vi "Test Read Strings.vi"(11 "TwinCAT ADS in":refnum<class "TwinCAT ADS.lvclass">) -> (3 "TwinCAT ADS out":refnum<class "TwinCAT ADS.lvclass">)   [LabVIEW 2018]
uses:
  TwinCAT ADS Class/TwinCAT ADS.lvclass
  da5912db-239c-466c-8894-2e4d3d3515d5.vi
  0b8e16e0-dc07-46b7-b0c9-e61de058ac04.vi
  9020aa95-6034-4dbf-83dd-b9edd1e76234.vi
  e5c40106-6d15-478c-83d1-da726149c43f.vi
  d432d6b6-cb13-4d15-9f79-374da6932203.vi
  66708433-c380-4caa-81db-290be98b0d9d.vi
  0e82c4fa-873b-4361-ac99-2e6e4b7cd392.vi
  da0f88be-82f8-4e5b-86e7-5baa69d9b51e.vi
  4782b519-43e7-4b8e-bd72-e209be860882.vi
  e7a7b24b-aede-49d7-b369-bb451e1de87e.vi
  TwinCAT ADS Class/VIs/Data/Read.vi
  <vilib>/addons/_JKI Toolkits/Caraya/classes/Assert/Assert Equal Value and Type_Variant.vi
  <vilib>/addons/_JKI Toolkits/Caraya/classes/Assert/Assert.lvclass
  <vilib>/addons/_JKI Toolkits/Caraya/classes/Test/Test.lvclass
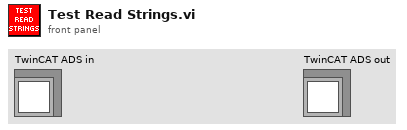
[diagram p1: front panel]
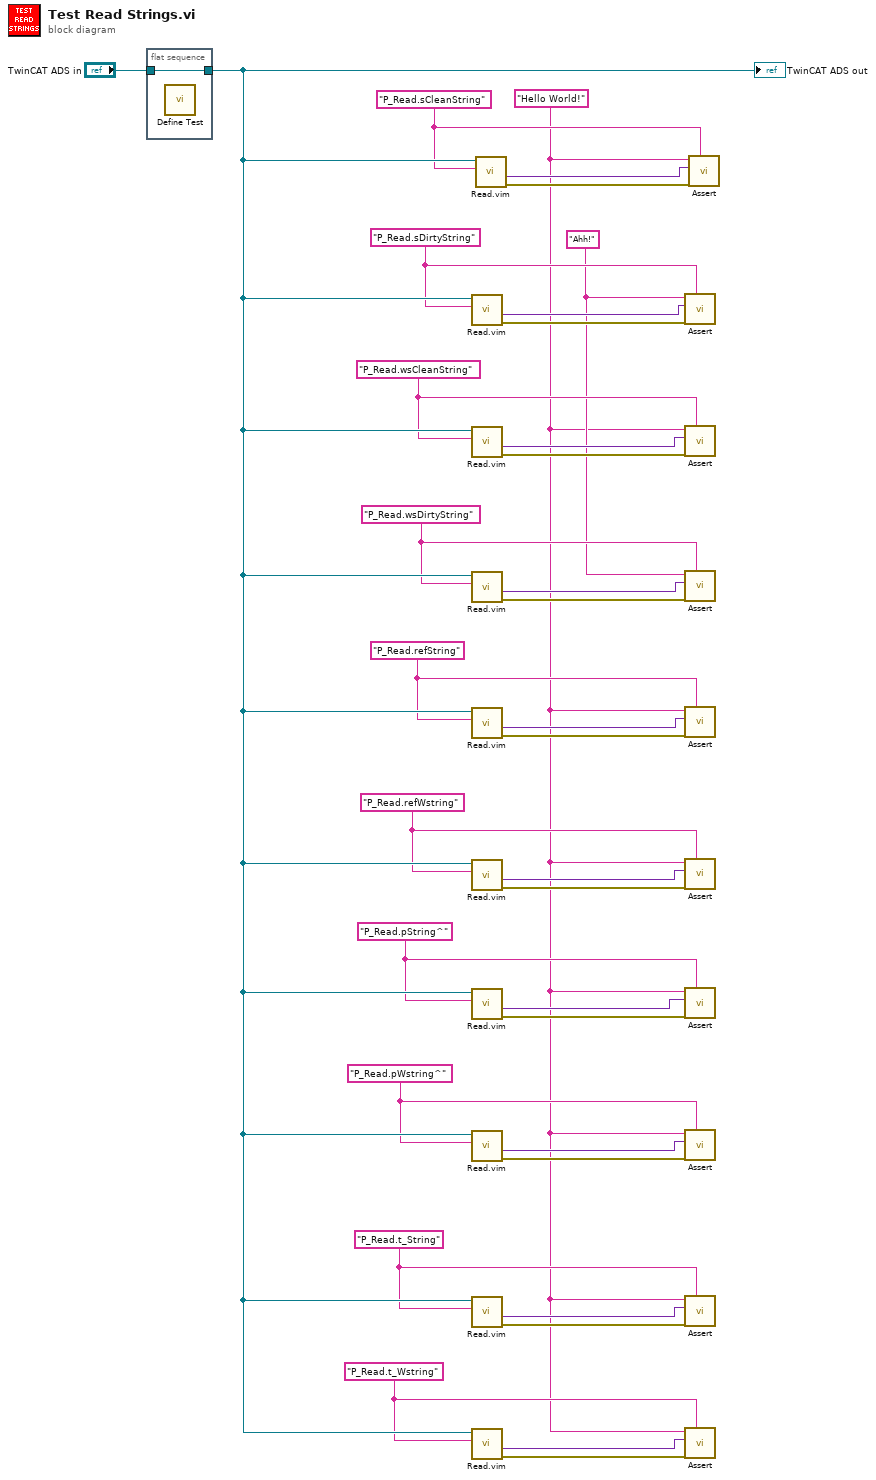
[diagram p0: block diagram]
diagram:
  w4 = "P_Read.t_Wstring" ("Symbol Name")
  w5 = "P_Read.t_String" ("Symbol Name")
  w8 = "Ahh!" ("Symbol Name")
  w1 = "Hello World!" ("Symbol Name")
  w16 = "P_Read.pWstring^" ("Symbol Name")
  w17 = "P_Read.pString^" ("Symbol Name")
  w20 = "P_Read.refWstring" ("Symbol Name")
  w21 = "P_Read.refString" ("Symbol Name")
  w26 = "P_Read.wsDirtyString" ("Symbol Name")
  w27 = "P_Read.wsCleanString" ("Symbol Name")
  w30 = "P_Read.sDirtyString" ("Symbol Name")
  w31 = "P_Read.sCleanString" ("Symbol Name")
  n1 = flat-sequence {
    tunnel: "TwinCAT ADS in" -> [w35]
    tunnel: [w35] -> w34
    frame #0 {
      n2 = call <vilib>:"Define Test.vi"() -> ()  [unwired: 10 in, 2 out]
    }
  }
  n3 = call "Read.vim"("Symbol Name"=w30, "TwinCAT ADS in"=w34) -> ("error out"=w29:errorcluster, "Value"=w23:variant)  [unwired: 7 in, 1 out]
  n4 = call "Read.vim"("Symbol Name"=w27, "TwinCAT ADS in"=w34) -> ("error out"=w28:errorcluster, "Value"=w12:variant)  [unwired: 7 in, 1 out]
  n5 = call "Read.vim"("Symbol Name"=w26, "TwinCAT ADS in"=w34) -> ("error out"=w25:errorcluster, "Value"=w13:variant)  [unwired: 7 in, 1 out]
  n6 = call "Read.vim"("Symbol Name"=w21, "TwinCAT ADS in"=w34) -> ("error out"=w22:errorcluster, "Value"=w14:variant)  [unwired: 7 in, 1 out]
  n7 = call "Read.vim"("Symbol Name"=w20, "TwinCAT ADS in"=w34) -> ("error out"=w19:errorcluster, "Value"=w11:variant)  [unwired: 7 in, 1 out]
  n8 = call "Read.vim"("Symbol Name"=w17, "TwinCAT ADS in"=w34) -> ("error out"=w18:errorcluster, "Value"=w10:variant)  [unwired: 7 in, 1 out]
  n9 = call "Read.vim"("Symbol Name"=w16, "TwinCAT ADS in"=w34) -> ("error out"=w15:errorcluster, "Value"=w9:variant)  [unwired: 7 in, 1 out]
  n10 = call "Read.vim"("Symbol Name"=w5, "TwinCAT ADS in"=w34) -> ("error out"=w6:errorcluster, "Value"=w7:variant)  [unwired: 7 in, 1 out]
  n11 = call "Read.vim"("Symbol Name"=w4, "TwinCAT ADS in"=w34) -> ("error out"=w3:errorcluster, "Value"=w2:variant)  [unwired: 7 in, 1 out]
  n12 = call "Read.vim"("Symbol Name"=w31, "TwinCAT ADS in"=w34) -> ("error out"=w33:errorcluster, "Value"=w24:variant)  [unwired: 7 in, 1 out]
  n13 = call-poly <vilib>:"Assert.vi"("Label"=w30, "error in (no error)"=w29, "Y"=w23, "X"=w8) -> ()  [unwired: 6 in, 2 out]
  n14 = call-poly <vilib>:"Assert.vi"("Label"=w27, "error in (no error)"=w28, "Y"=w12, "X"=w1) -> ()  [unwired: 6 in, 2 out]
  n15 = call-poly <vilib>:"Assert.vi"("Label"=w26, "error in (no error)"=w25, "Y"=w13, "X"=w8) -> ()  [unwired: 6 in, 2 out]
  n16 = call-poly <vilib>:"Assert.vi"("Label"=w21, "error in (no error)"=w22, "Y"=w14, "X"=w1) -> ()  [unwired: 6 in, 2 out]
  n17 = call-poly <vilib>:"Assert.vi"("Label"=w20, "error in (no error)"=w19, "Y"=w11, "X"=w1) -> ()  [unwired: 6 in, 2 out]
  n18 = call-poly <vilib>:"Assert.vi"("Label"=w17, "error in (no error)"=w18, "Y"=w10, "X"=w1) -> ()  [unwired: 6 in, 2 out]
  n19 = call-poly <vilib>:"Assert.vi"("Label"=w16, "error in (no error)"=w15, "Y"=w9, "X"=w1) -> ()  [unwired: 6 in, 2 out]
  n20 = call-poly <vilib>:"Assert.vi"("Label"=w5, "error in (no error)"=w6, "Y"=w7, "X"=w1) -> ()  [unwired: 6 in, 2 out]
  n21 = call-poly <vilib>:"Assert.vi"("Label"=w4, "error in (no error)"=w3, "Y"=w2, "X"=w1) -> ()  [unwired: 6 in, 2 out]
  n22 = call-poly <vilib>:"Assert.vi"("Label"=w31, "error in (no error)"=w33, "Y"=w24, "X"=w1) -> ()  [unwired: 6 in, 2 out]
  "TwinCAT ADS out" <- w34
